vi "Wrap String Parameters in Quotes.vi"(1 "Optimise parameter - string in":T1) -> (0 "Optimise parameter - string out":T1)   [LabVIEW 2020, in "TALOS.lvlib" / "Run Utilities.lvlib" / "Optimiser SBlock.lvclass"]
doc: "VI for wrapping strings in the \\\" marks (the backslash is to allow the string to be passed inside a longer string)"
uses:
  Optimiser SBlock.lvclass
  Optimiser Cell/Optimise parameter - string.ctl
  Optimiser SBlock.lvclass/Optimiser SBlock.ctl
  Run Utilities.lvlib
  Optimiser Cell/Optimiser Cell.lvclass
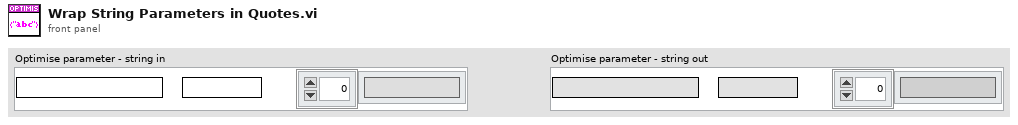
[diagram p1: front panel]
types:
  T1 = typedef "TALOS.lvlib/Run Utilities.lvlib/Optimiser Cell.lvclass/Optimise parameter - string.ctl" = cluster{"Name":string, "Start value":string, "Options":string[]}
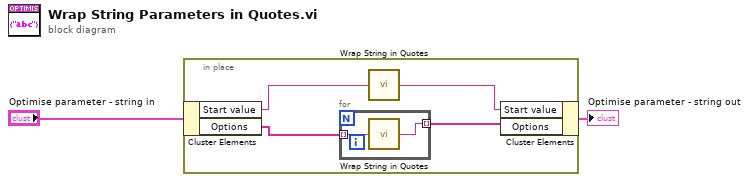
[diagram p0: block diagram]
diagram:
  n1 = in-place {
    n2 = in-place-cluster #1("Optimise parameter - string in") -> ("Start value"=w6:string, "Options"=w4:string[])
    n3 = for {
      tunnel: w4 -> [w8] mode=indexing
      tunnel: [w7] -> w3 mode=indexing
      n4 = call "Wrap String in Quotes.vi"("String in"=w8) -> ("String out"=w7:string)
    }
    n5 = call "Wrap String in Quotes.vi"("String in"=w6) -> ("String out"=w5:string)
    n6 = in-place-cluster #1("Start value"=w5, "Options"=w3) -> (→"Optimise parameter - string out":T1)
  }
